vi "Tip tune ZaberAndSR865 Static.vi"(0 "Z axis":T3={"Serial port handle"="", "Axis"="", "Controller #"=0, "Min position"=0.0, "Max position"=0.0, "Min velocity"=0.0, "Max velocity"=0.0, "Firmware"="", "Device ID"=0, "Variable event"=refnum, "Variable ref"=refnum, "Resolution, usteps/step"=0, "Serial port semaphore"=refnum, "Joystick buttons"={"MinDir"=1, "MaxDir"=2, "MedSpeed"=5, "HighSpeed"=6}} {"Joystick buttons"."HighSpeed" min=1 max=25 step=1; "Joystick buttons"."MedSpeed" min=1 max=25 step=1; "Joystick buttons"."MaxDir" min=1 max=25 step=1; "Joystick buttons"."MinDir" min=1 max=25 step=1}, 1 "SR865":T1, 5 "error in":errorcluster) -> (19 "error out":errorcluster)   [LabVIEW 2018]
uses:
  Zaber library/Zaber.ctl
  GenericDataEvent/GenericEvent.ctl
  Zaber library/ZaberVariables.ctl
  SR865/SR865.ctl
  SR865/OutSineReference.ctl
  SR865/OutSineSource.ctl
  SR865/DataChannel.ctl
  <vilib>/Analysis/6fits.llb/Curve Fitting Criteria.ctl
  <vilib>/Analysis/NI_AAL_SigProc.lvlib
  <vilib>/Analysis/NI_AALBase.lvlib
  <vilib>/Analysis/NI_AALPro.lvlib
panel:
  in  "BtnQuit":bool
  in  "btnReadSignal":bool
  out "Signal":dbl=100000.0 caption="Signal, mV"
  in  "BtnZ-":bool
  in  "BtnZ+":bool
  in  "ZStep":dbl=0.005 caption="Z step, mm" min=0.0 max=25.0 step=0.01 format="%#.4f"
  in  "btnStartPosScanning":bool caption="stop"
  in  "btnCalculateSlope":bool
  in  "btnCalculateSurfaceLevel":bool
  in  "btnCalculateAirLevel":bool
  out "FrequencyStepRb":dbl=100000.0 caption="Frequency"
  out "PhaseRb":dbl=100000.0 caption="Frequency"
  out "AmplitudeRb":dbl=100000.0 caption="Frequency"
  out "DCOffsetRb":dbl=100000.0 caption="DC offset, V"
  out "SlopeError":dbl=8.6 caption="Slope error, V/mm" min=0.0 max=25.0 step=0.01 format="%#.4f"
  out "SurfaceError":dbl=8.6 caption="Surface error, V" min=0.0 max=25.0 step=0.01 format="%#.4f"
  out "AirError":dbl=8.6 caption="Air error, V" min=0.0 max=25.0 step=0.01 format="%#.4f"
  out "Slope":dbl=8.6 caption="Slope, mm/V" min=0.0 max=25.0 step=0.01 format="%#.4f"
  out "SurfaceLevel":dbl=8.6 caption="Surface level, V" min=0.0 max=25.0 step=0.01 format="%#.4f"
  out "AirLevel":dbl=8.6 caption="Air level, V" min=0.0 max=25.0 step=0.01 format="%#.4f"
  out "CurrentStep":i32=61 caption="Z steps"
  out "PltScanningPosition":cluster{dbl[], dbl[]}[](graph) caption="Position scanning"
  out "ZStep":dbl=0.0016666666666666607 caption="Z step, mm" min=0.0 max=25.0 format="%#.4f"
  in  "Frequency":dbl=97044.98 caption="Frequency, Hz" format="%.2p"
  in  "BtnSetZEndPosition":bool
  in  "BtnSetZStartPosition":bool
  in  "ZPoints":i32=61 caption="Z points"
  out "ZEndPosition":dbl=8.6 caption="Z end, mm" min=0.0 max=25.0 format="%#.4f"
  out "ZStartPosition":dbl=8.5 caption="Z start, mm" min=0.0 max=25.0 format="%#.4f"
  out "ZPositionRb":dbl=8.6 caption="Z position" min=0.0 max=25.0 step=0.01 format="%#.4f"
  in  "ZPosition":dbl=8.5 caption="Z position, mm" min=0.0 max=25.0 step=0.01 format="%#.4f"
  out "TblBestFrequencyies":string[][](table)=[["97044.98", "2.85"], ["82864.39", "1.68"], ["21141.21", "1.26"], ["93904.03", "0.82"], ["15778.11", "0.52"]] caption="Best frequencies, Hz"
  in  "TipPlace":u16(ring)=1 caption="Tip place" items=["Air", "Surface"]
  in  "SettingTime":u32=1000 caption="Setting time, ms"
  out "FrequencyRb":dbl=100000.0 caption="Frequency"
  out "CurrentPoint":i32=90
  out "PltScanningFrequence":cluster{dbl[], dbl[]}[](graph)=[{[10000.0, 11000.0, 12000.0, 13000.0, 14000.0, 15000.0, 16000.0, 17000.0, 18000.0, 19000.0, 20000.0, 21000.0, 22000.0, 23000.0, 24000.0, 25000.0, 26000.0, 27000.0, 28000.0, 29000.0, 30000.0, 31000.0, 32000.0, 33000.0, 34000.0, 35000.0, 36000.0, 37000.0, 38000.0, 39000.0, 40000.0, 41000.0, 42000.0, 43000.0, 44000.0, 45000.0, 46000.0, 47000.0, 48000.0, 49000.0, 50000.0, 51000.0, 52000.0, 53000.0, 54000.0, 55000.0, 56000.0, 57000.0, 58000.0, 59000.0, 60000.0, 61000.0, 62000.0, 63000.0, 64000.0, 65000.0, 66000.0, 67000.0, 68000.0, 69000.0, 70000.0, 71000.0, 72000.0, 73000.0, 74000.0, 75000.0, 76000.0, 77000.0, 78000.0, 79000.0, 80000.0, 81000.0, 82000.0, 83000.0, 84000.0, 85000.0, 86000.0, 87000.0, 88000.0, 89000.0, 90000.0, 91000.0, 92000.0, 93000.0, 94000.0, 95000.0, 96000.0, 97000.0, 98000.0, 99000.0, 100000.0], [3.5655190000512516, 3.4374305005139005, 3.4273711461139715, 3.4850248112142093, 3.5761130550998383, 3.556590231281875, 3.5082421792498932, 3.012145327734691, 3.60479334690102, 3.6237170567298436, 3.5213679819034964, 4.863866373270507, 4.004233765623082, 3.958662171251218, 3.638372868429504, 3.6863311988676024, 3.6407628928169347, 3.597268956374069, 3.472475578654757, 3.4138362740831423, 4.023460288827825, 3.8711427099095466, 3.8072787456116726, 3.773067870768127, 3.802872335674139, 3.843425482975206, 3.8131604010931146, 3.710485915669144, 3.68892415072003, 3.7175819077370553, 3.6497045488279003, 3.698426272759254, 3.738228894609222, 3.7572105957332433, 3.841541162636644, 3.552982648310411, 3.6359506328697484, 3.7367182179969376, 3.817937233155462, 3.940743403433729, 4.337961900873752, 3.232249392203631, 3.031809835447508, 3.1009883283630275, 3.1785447948663723, 2.9738534939166783, 3.794967857187948, 3.786370846678634, 3.691365712894553, 3.655859990170908, 3.6562916119155986, 3.5957679438322634, 3.593065477052433, 3.5925726553448727, 3.5922634338806207, 3.590250273321926, 3.597758557035468, 3.5946888897478324, 3.606027010467748, 3.573291409437125, 3.5650938203985896, 3.532467740941366, 3.385655269781037, 3.651862657728945, 3.6418741576807374, 3.5802843235408948, 3.611222575631784, 3.5164236610651676, 4.632535226763082, 3.2424697969441687, 3.272032610844888, 3.3549199729897623, 3.7972193768166784, 5.452081044437504, 2.748058067103696, 2.9130046647694234, 2.9576226283303546, 3.0336329490386387, 3.0499346821806705, 2.9810010016675736, 2.8330872460617447, 2.3801761264752517, 1.3887019949256822, 6.48560906859755, 5.721885978735551, 3.7523307011355125, 2.996072291328326, 5.390088024437564, 5.438011320322094, 4.595058047439225, 4.5440910275334865]}, {[10000.0, 11000.0, 12000.0, 13000.0, 14000.0, 15000.0, 16000.0, 17000.0, 18000.0, 19000.0, 20000.0, 21000.0, 22000.0, 23000.0, 24000.0, 25000.0, 26000.0, 27000.0, 28000.0, 29000.0, 30000.0, 31000.0, 32000.0, 33000.0, 34000.0, 35000.0, 36000.0, 37000.0, 38000.0, 39000.0, 40000.0, 41000.0, 42000.0, 43000.0, 44000.0, 45000.0, 46000.0, 47000.0, 48000.0, 49000.0, 50000.0, 51000.0, 52000.0, 53000.0, 54000.0, 55000.0, 56000.0, 57000.0, 58000.0, 59000.0, 60000.0, 61000.0, 62000.0, 63000.0, 64000.0, 65000.0, 66000.0, 67000.0, 68000.0, 69000.0, 70000.0, 71000.0, 72000.0, 73000.0, 74000.0, 75000.0, 76000.0, 77000.0, 78000.0, 79000.0, 80000.0, 81000.0, 82000.0, 83000.0, 84000.0, 85000.0, 86000.0, 87000.0, 88000.0, 89000.0, 90000.0, 91000.0, 92000.0, 93000.0, 94000.0, 95000.0, 96000.0, 97000.0, 98000.0, 99000.0, 100000.0], [3.6968028657407785, 3.397109339181018, 3.567193952093816, 3.4622519508906793, 3.5945342790368535, 3.5386940424582525, 3.029648511216874, 3.7294031949868516, 3.854496267967221, 3.66608362794549, 3.6337442084525384, 3.622335223134029, 3.520269601833684, 3.625449985669437, 3.5996783070122036, 3.596367060420739, 3.6706800775467205, 3.6178547324397927, 3.494530145248237, 3.4783507835572123, 3.9798696462301795, 3.909521653058709, 3.84636309009401, 3.8283541416529783, 3.8855956102501024, 3.948232372330415, 3.8955390259265563, 3.7044271046719377, 3.6476140823855085, 3.685313344462496, 3.639751480735465, 3.690521795627914, 3.727960158953497, 3.75535848669949, 3.8145229094921054, 3.5935582988975963, 3.6440902453414807, 3.730672290482194, 3.7940627371494946, 3.884890197869988, 4.123519414820418, 5.233578709141258, 2.8898807738384256, 2.709737263826195, 3.650699858167375, 3.6058691787236263, 3.5725795559217843, 3.585563635600408, 3.5978873993164835, 3.6012115301523817, 3.545358407800998, 3.557833559064785, 3.5697611313701043, 3.5699866053317777, 3.5644109564113067, 3.568540350922504, 3.570524521787714, 3.5653418417511418, 3.5472878205078633, 3.566549737959607, 3.5284381997956884, 3.443283156254747, 3.726391503493266, 3.6588555739683373, 3.5487920538102036, 3.744426212291304, 3.774333747133092, 3.7278280955270975, 4.291694487008893, 3.381445353898666, 3.4274420088262834, 3.5326255726860984, 3.8970271568359123, 3.8148611207822927, 4.140697353288415, 3.4812175242568655, 3.7482206201906454, 2.959581027358073, 2.755453572987086, 2.842289778548217, 2.8230407994627473, 2.5397852639697267, 1.7720535165304037, 6.311279502338936, 4.911483553972613, 3.8801745664846505, 3.1735908186482717, 2.5479667164400683, 5.117117280660982, 5.956381695510879, 6.236143926446963]}, {[10000.0, 11000.0, 12000.0, 13000.0, 14000.0, 15000.0, 16000.0, 17000.0, 18000.0, 19000.0, 20000.0, 21000.0, 22000.0, 23000.0, 24000.0, 25000.0, 26000.0, 27000.0, 28000.0, 29000.0, 30000.0, 31000.0, 32000.0, 33000.0, 34000.0, 35000.0, 36000.0, 37000.0, 38000.0, 39000.0, 40000.0, 41000.0, 42000.0, 43000.0, 44000.0, 45000.0, 46000.0, 47000.0, 48000.0, 49000.0, 50000.0, 51000.0, 52000.0, 53000.0, 54000.0, 55000.0, 56000.0, 57000.0, 58000.0, 59000.0, 60000.0, 61000.0, 62000.0, 63000.0, 64000.0, 65000.0, 66000.0, 67000.0, 68000.0, 69000.0, 70000.0, 71000.0, 72000.0, 73000.0, 74000.0, 75000.0, 76000.0, 77000.0, 78000.0, 79000.0, 80000.0, 81000.0, 82000.0, 83000.0, 84000.0, 85000.0, 86000.0, 87000.0, 88000.0, 89000.0, 90000.0, 91000.0, 92000.0, 93000.0, 94000.0, 95000.0, 96000.0, 97000.0, 98000.0, 99000.0, 100000.0], [-0.131283865689527, 0.04032116133288266, -0.1398228059798443, 0.022772860323529986, -0.018421223937015174, 0.017896188823622428, 0.47859366803301917, -0.7172578672521608, -0.24970292106620118, -0.04236657121564624, -0.112376226549042, 1.2415311501364776, 0.4839641637893983, 0.3332121855817811, 0.03869456141730021, 0.08996413844686346, -0.029917184729785884, -0.02058577606572376, -0.02205456659347993, -0.06451450947407, 0.043590642597645335, -0.03837894314916257, -0.03908434448233722, -0.05528627088485116, -0.0827232745759634, -0.10480688935520899, -0.08237862483344172, 0.0060588109972061766, 0.04131006833452133, 0.03226856327455918, 0.009953068092435124, 0.007904477131339682, 0.01026873565572517, 0.0018521090337535462, 0.02701825314453865, -0.04057565058718504, -0.008139612471732338, 0.006045927514743532, 0.023874496005967583, 0.05585320556374107, 0.2144424860533345, -2.0013293169376274, 0.14192906160908247, 0.39125106453683234, -0.47215506330100254, -0.632015684806948, 0.2223883012661636, 0.2008072110782262, 0.09347831357806946, 0.05464846001852619, 0.1109332041146005, 0.037934384767478235, 0.02330434568232853, 0.022586050013094994, 0.027852477469314074, 0.021709922399422155, 0.02723403524775403, 0.029347047996690634, 0.05873918995988481, 0.006741671477517919, 0.03665562060290117, 0.08918458468661905, -0.3407362337122293, -0.006992916239392244, 0.09308210387053384, -0.16414188875040914, -0.16311117150130805, -0.2114044344619299, 0.3408407397541886, -0.13897555695449748, -0.15540939798139553, -0.17770559969633615, -0.09980778001923385, 1.6372199236552114, -1.392639286184719, -0.568212859487442, -0.7905979918602908, 0.07405192168056551, 0.2944811091935846, 0.13871122311935657, 0.010046446598997338, -0.15960913749447503, -0.3833515216047214, 0.1743295662586144, 0.8104024247629376, -0.12784386534913805, -0.17751852731994555, 2.842121307997496, 0.32089403966111174, -1.3613236480716537, -1.6920528989134764]}] caption="Frequence scanning"
  in  "btnStartFreqScanning":bool caption="stop"
  out "FrequencyPoints":i32=91 caption="Frequency points"
  in  "FrequencyStep":dbl=1000.0 caption="Frequency step, Hz"
  in  "EndFrequency":dbl=100000.0 caption="End frequency, Hz" format="%.2p"
  in  "Phase":dbl format="%.3f"
  in  "StartFrequency":dbl=10000.0 caption="Start frequency, Hz" format="%.2p"
  in  "Amplitude":dbl=0.5 caption="Amplitude p-p, V" min=0.0 max=10.0 format="%.3f"
  # "RS865 parameters"
  # "Z stage parameters"
  # "Scanning parameters"
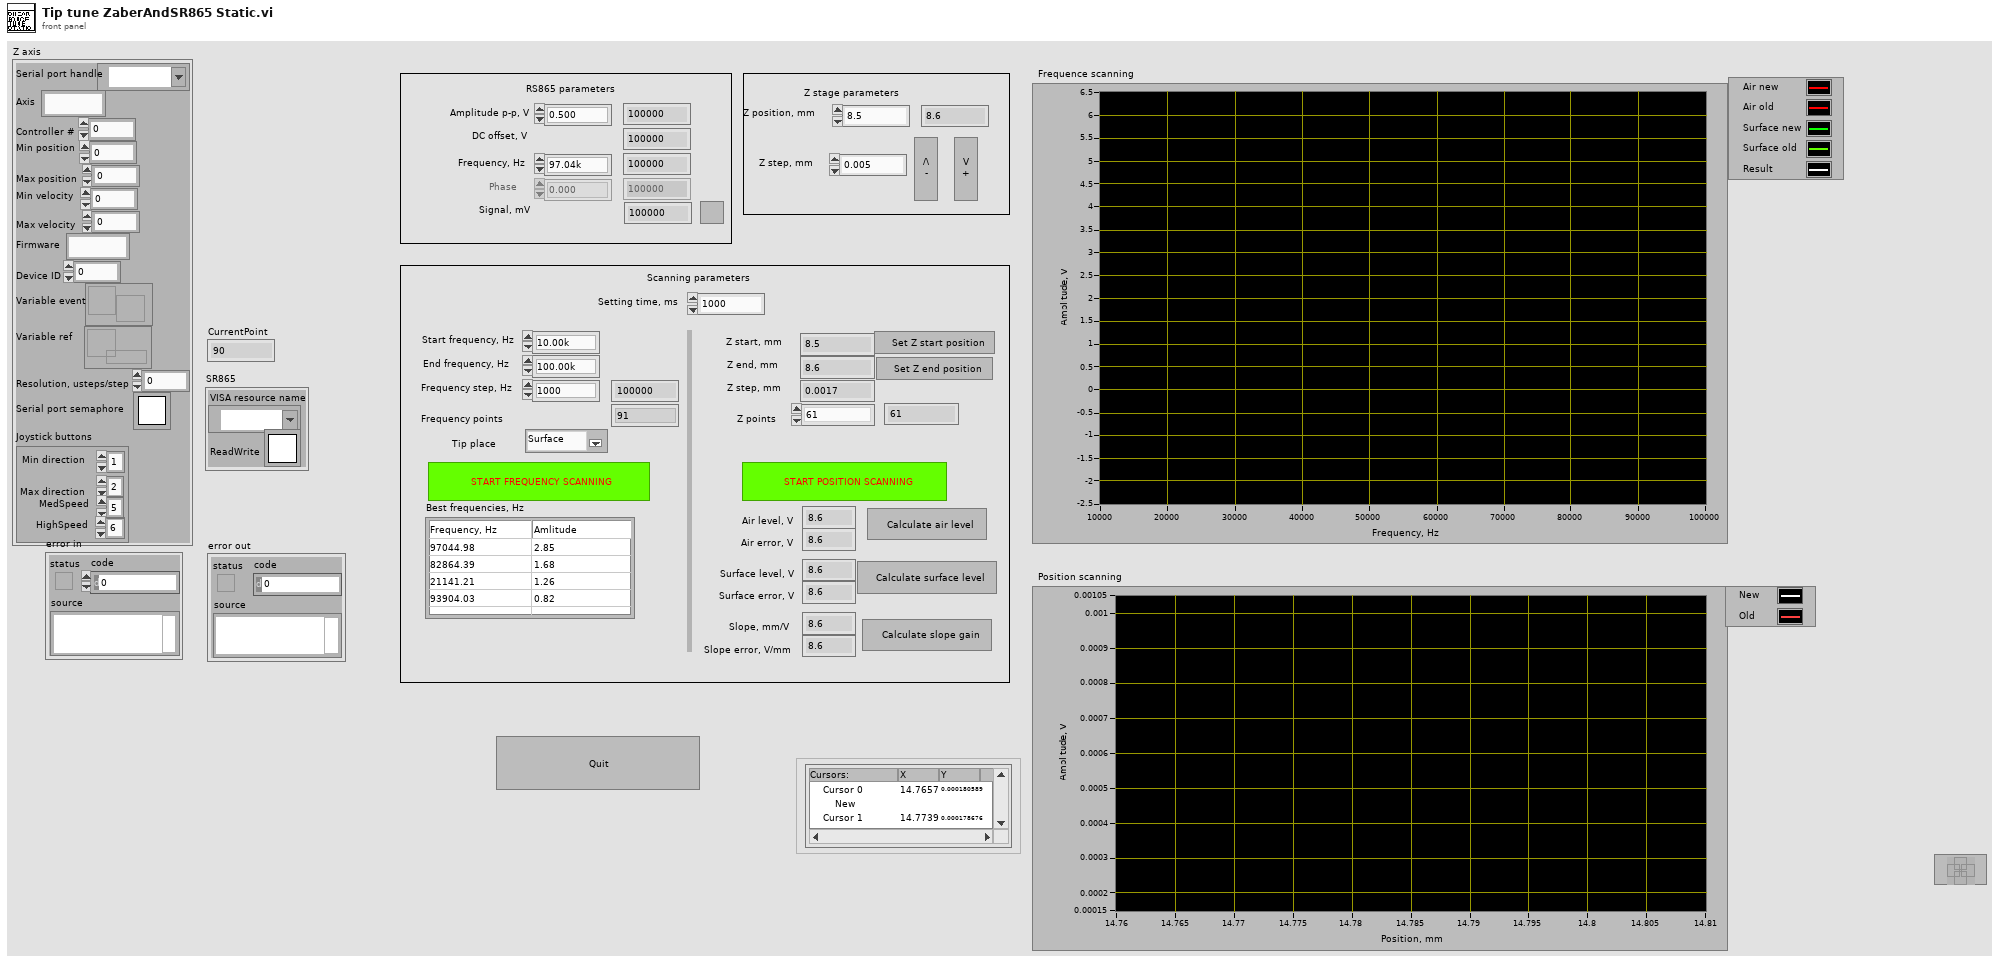
[diagram p1: front panel]
types:
  T1 = typedef "SR865.ctl" = cluster{"VISA resource name":refnum<visa-resource-name>, "ReadWrite":T2}
  T2 = typedef "Semaphore RefNum" = refnum<k1>
  T3 = typedef "Zaber.ctl" = cluster{"Serial port handle":refnum<visa-resource-name>, "Axis":string, "Controller #":u8, "Min position":dbl, "Max position":dbl, "Min velocity":dbl, "Max velocity":dbl, "Firmware":string, "Device ID":i32, "Variable event":T4, "Variable ref":refnum<data-value>, "Resolution, usteps/step":i32, "Serial port semaphore":T2, "Joystick buttons":cluster{"MinDir":i32, "MaxDir":i32, "MedSpeed":i32, "HighSpeed":i32}}
  T4 = typedef "GenericEvent.ctl" = refnum<user-event>
  T5 = typedef "DataChannel.ctl" = u16
  T6 = typedef "OutSineSource.ctl" = u16
  T7 = typedef "OutSineReference.ctl" = u16
  T8 = typedef "LVCursorListTypeDef.ctl" = cluster{"Name":string, "Color":u32, "Style":u8, "Point Style":u8, "Name Visible":bool, "Allow Drag":bool, "Cursor Mode":u32, "Plot":i32, "Index":i32, "Position":cluster{"X":dbl, "Y":dbl}, "X Scale":u32, "Y Scale":u32, "Watch Plots":i32[], "Watch All Plots":bool, "Plot Area":i32, "Label Offset":cluster{"X":dbl, "Y":dbl}}[]
  T9 = cluster{"Name":string, "Color":u32, "Style":u8, "Point Style":u8, "Name Visible":bool, "Allow Drag":bool, "Cursor Mode":u32, "Plot":i32, "Index":i32, "Position":cluster{"X":dbl, "Y":dbl}, "X Scale":u32, "Y Scale":u32, "Watch Plots":i32[], "Watch All Plots":bool, "Plot Area":i32, "Label Offset":cluster{"X":dbl, "Y":dbl}}
  T10 = typedef "NI_AALPro.lvlib/Curve Fitting Criteria.ctl" = u16
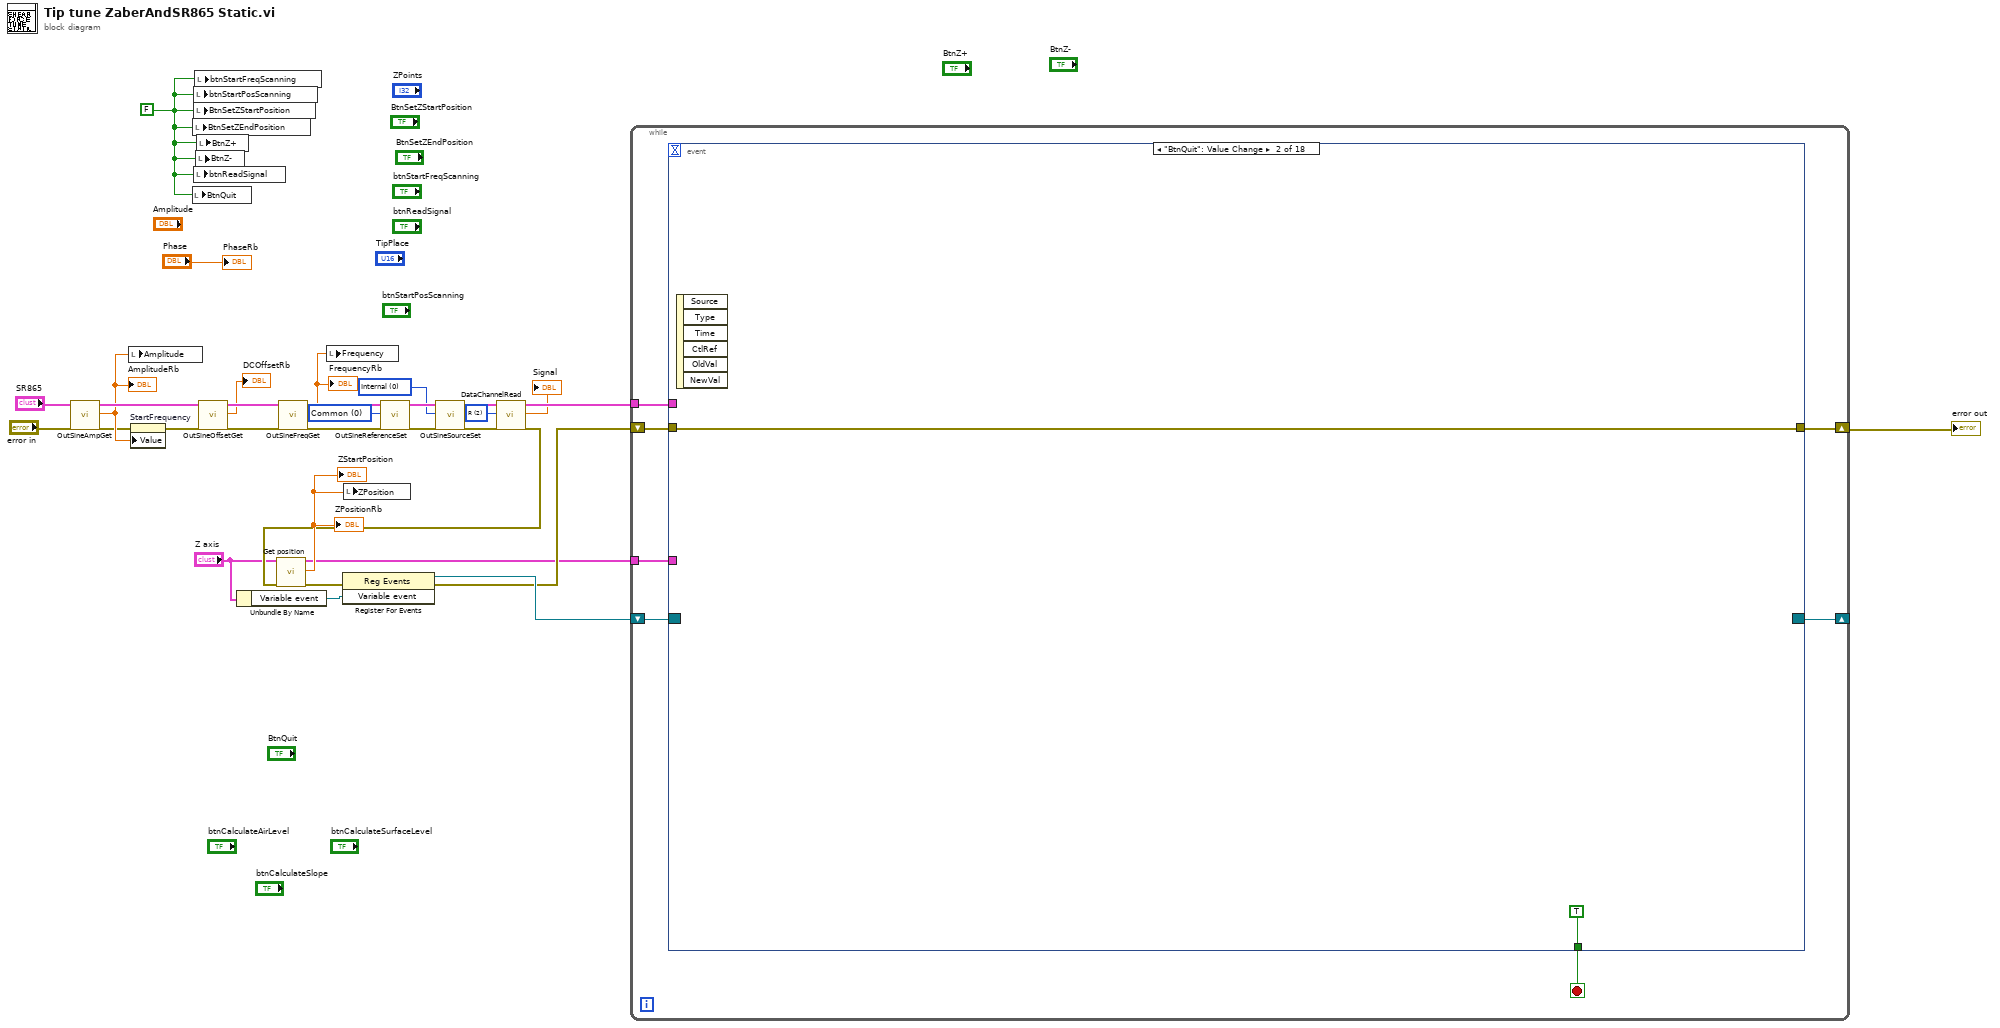
[diagram p0: block diagram]
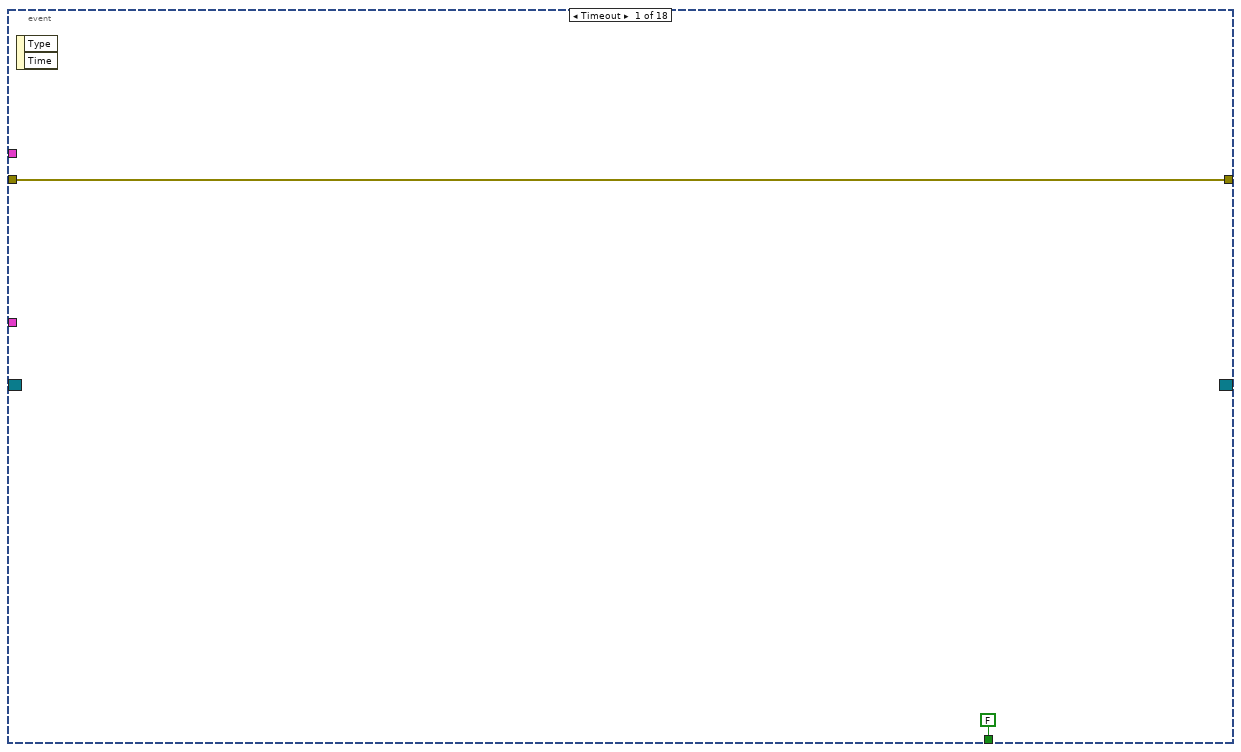
[diagram p2: hidden frame]
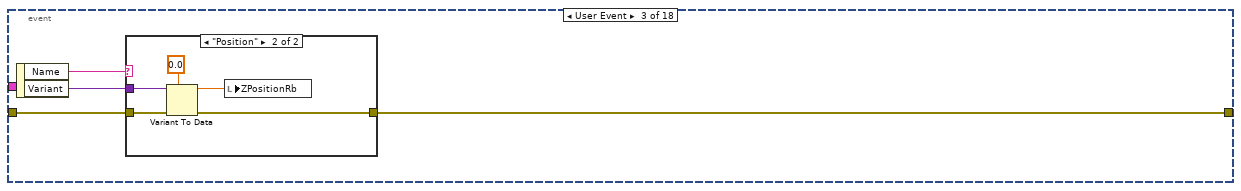
[diagram p3: hidden frame]
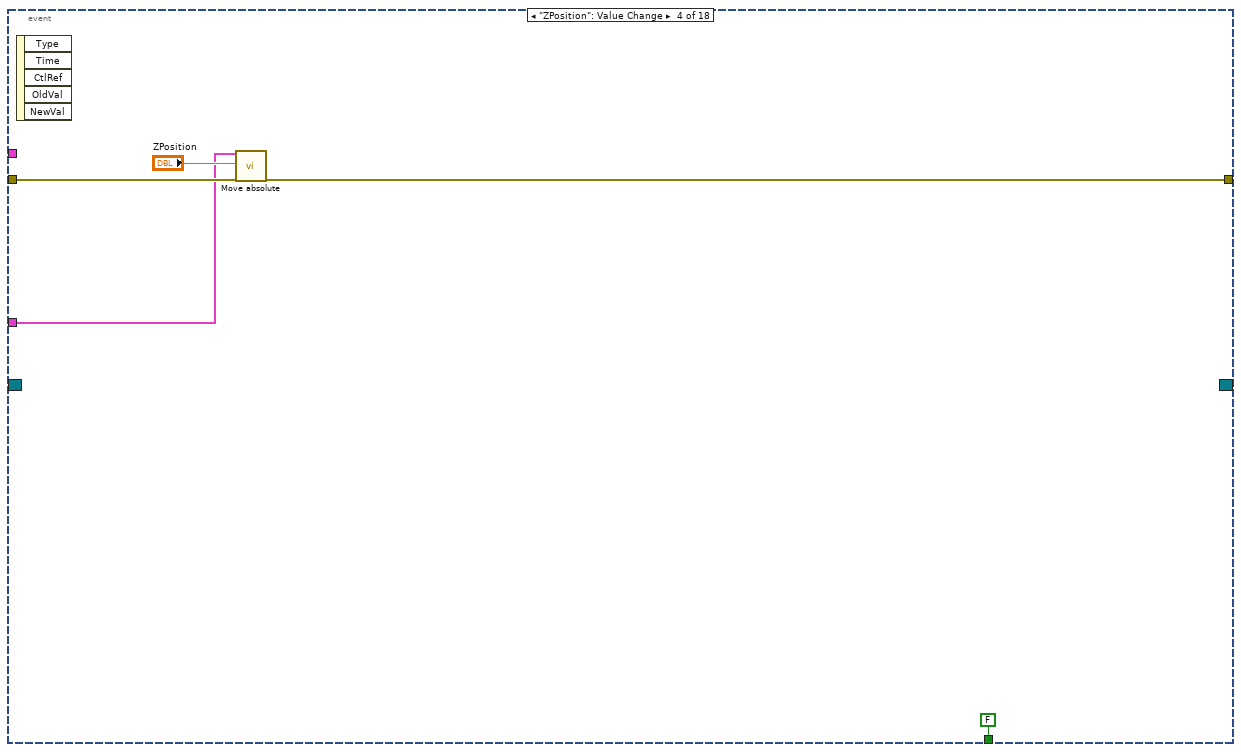
[diagram p5: hidden frame]
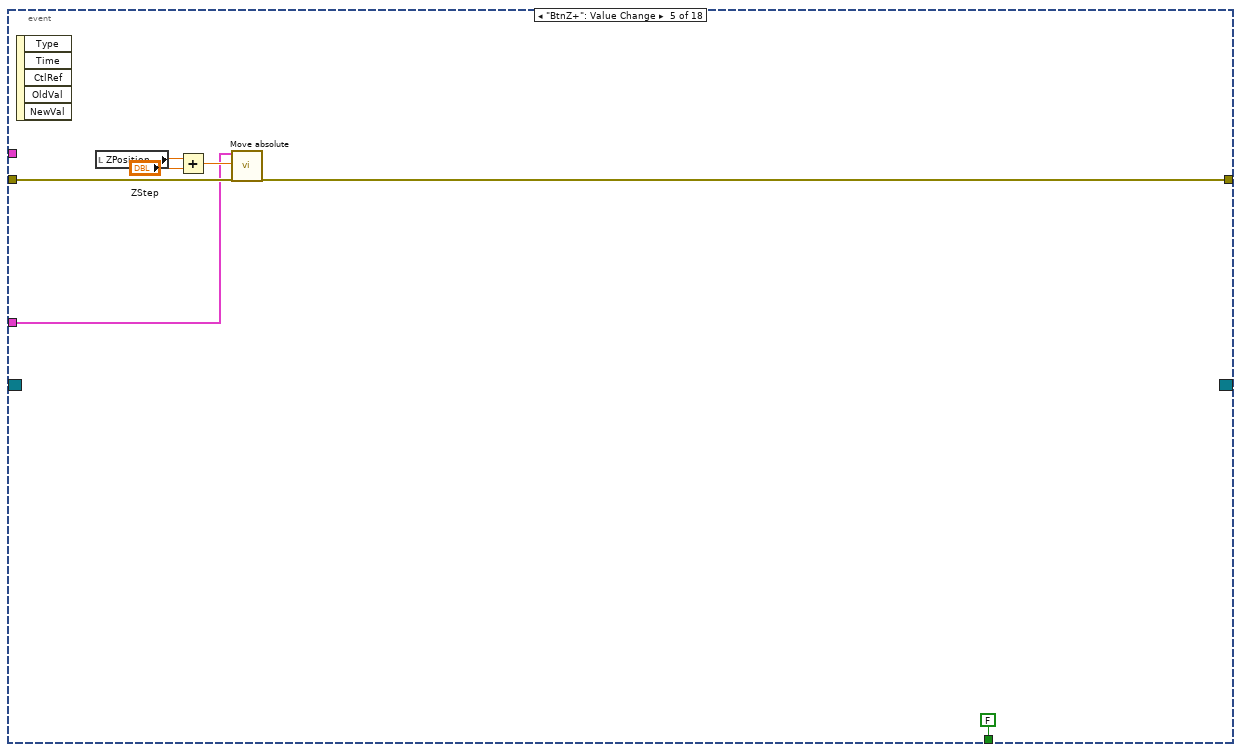
[diagram p6: hidden frame]
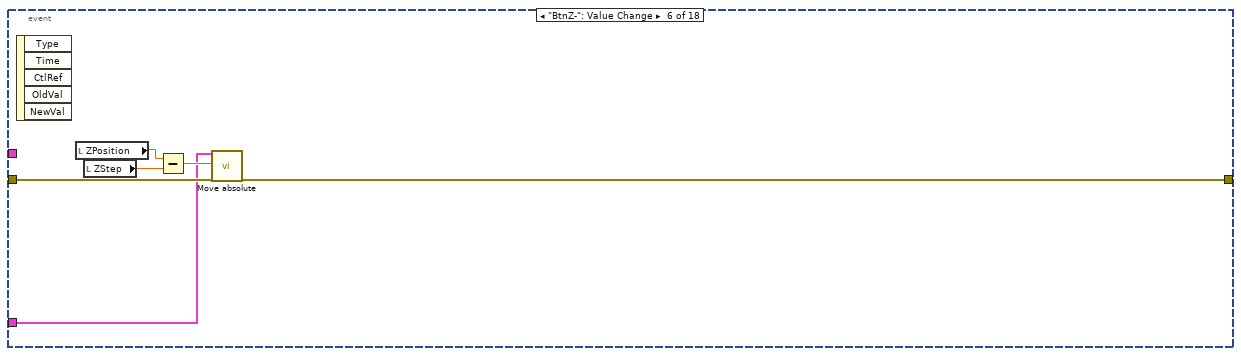
[diagram p7: hidden frame]
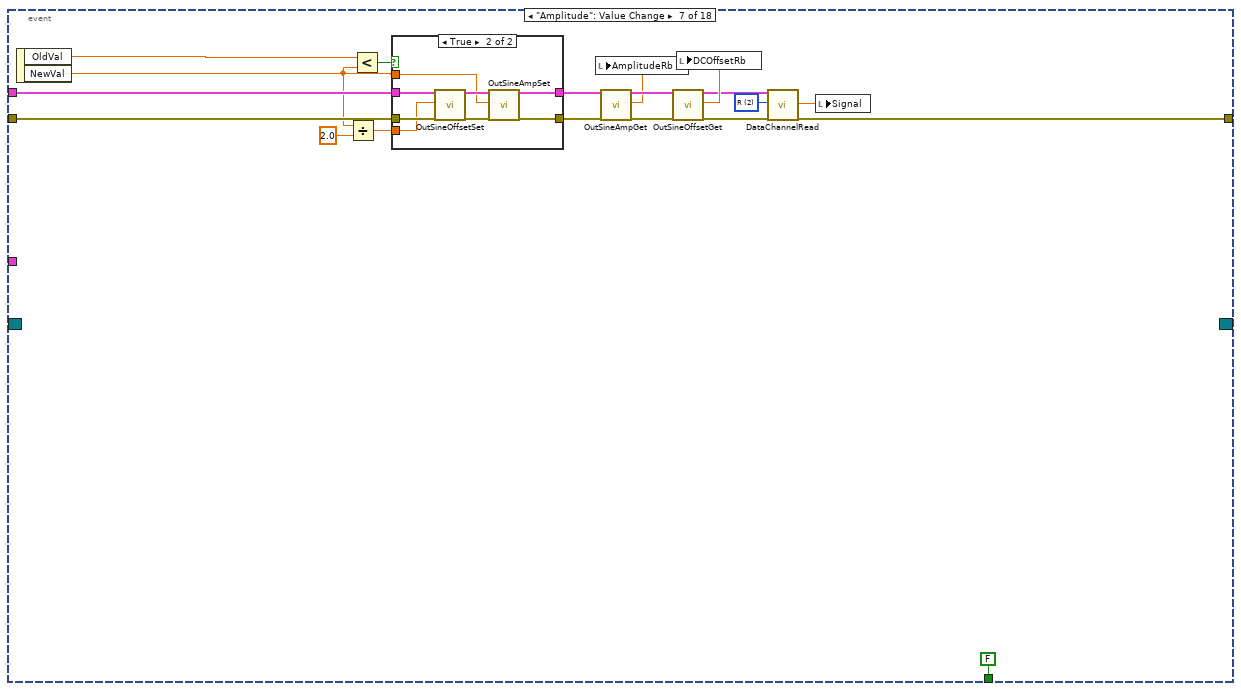
[diagram p8: hidden frame]
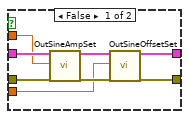
[diagram p9: hidden frame]
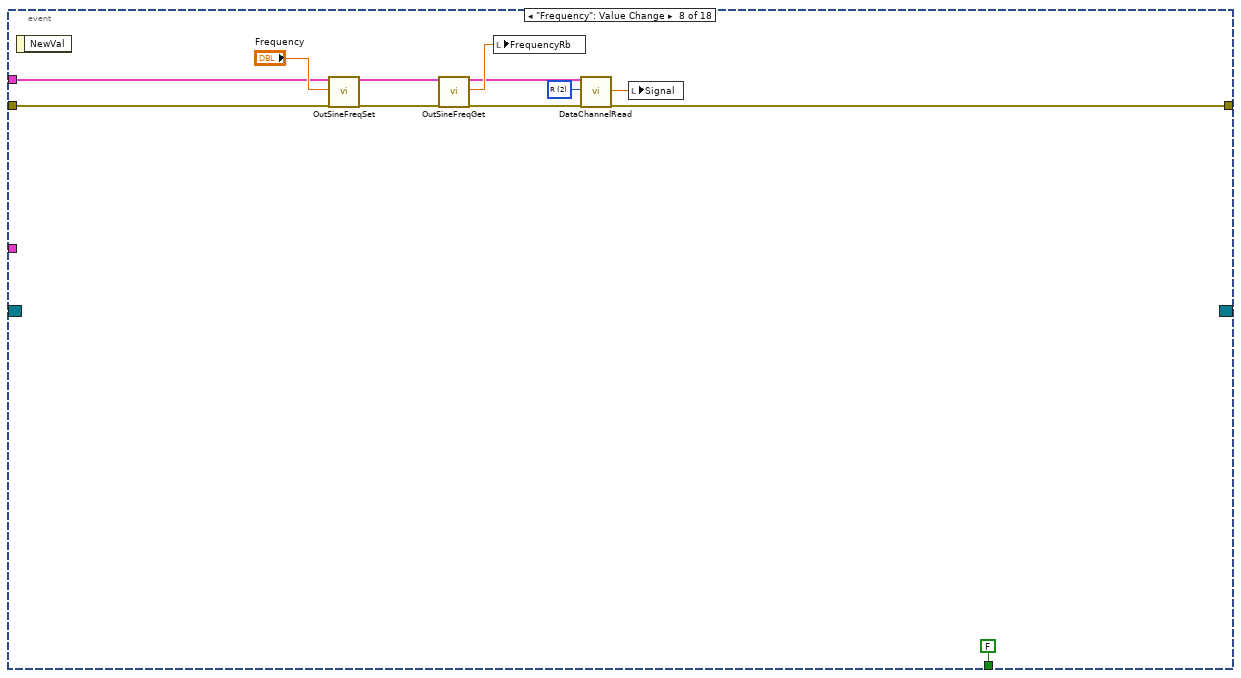
[diagram p10: hidden frame]
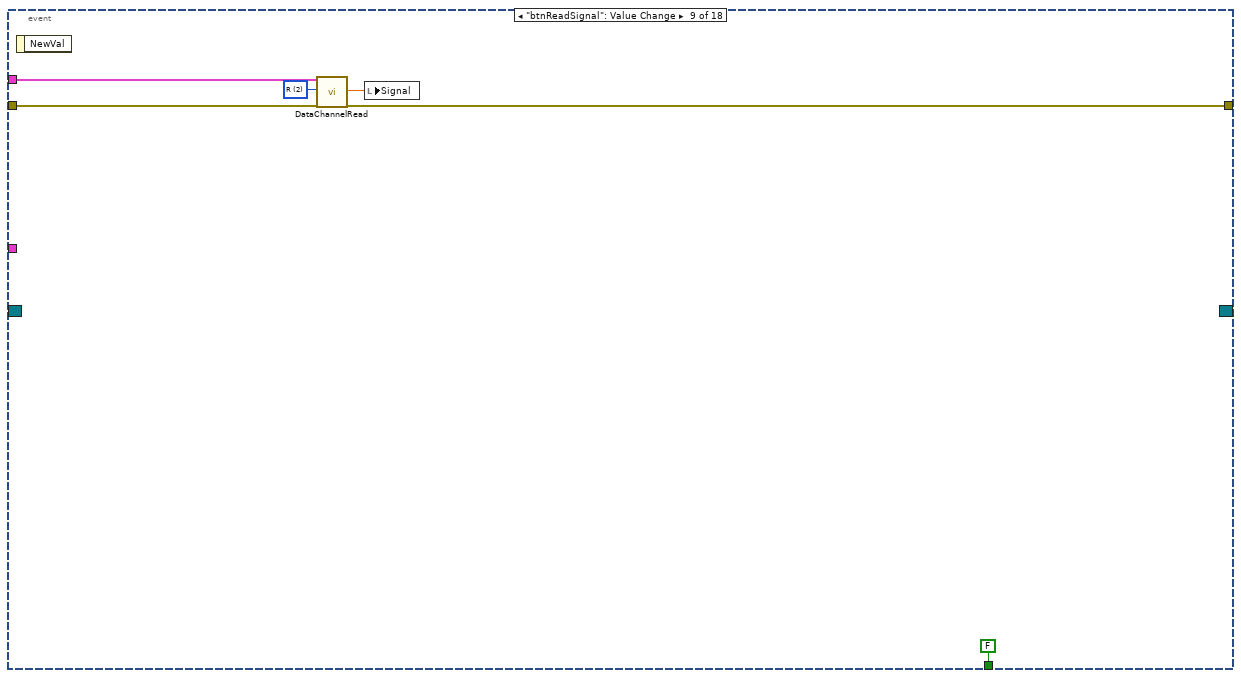
[diagram p11: hidden frame]
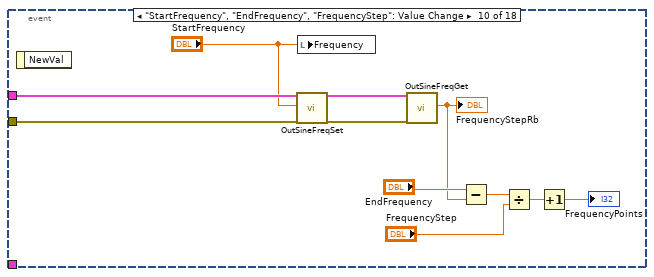
[diagram p12: hidden frame]
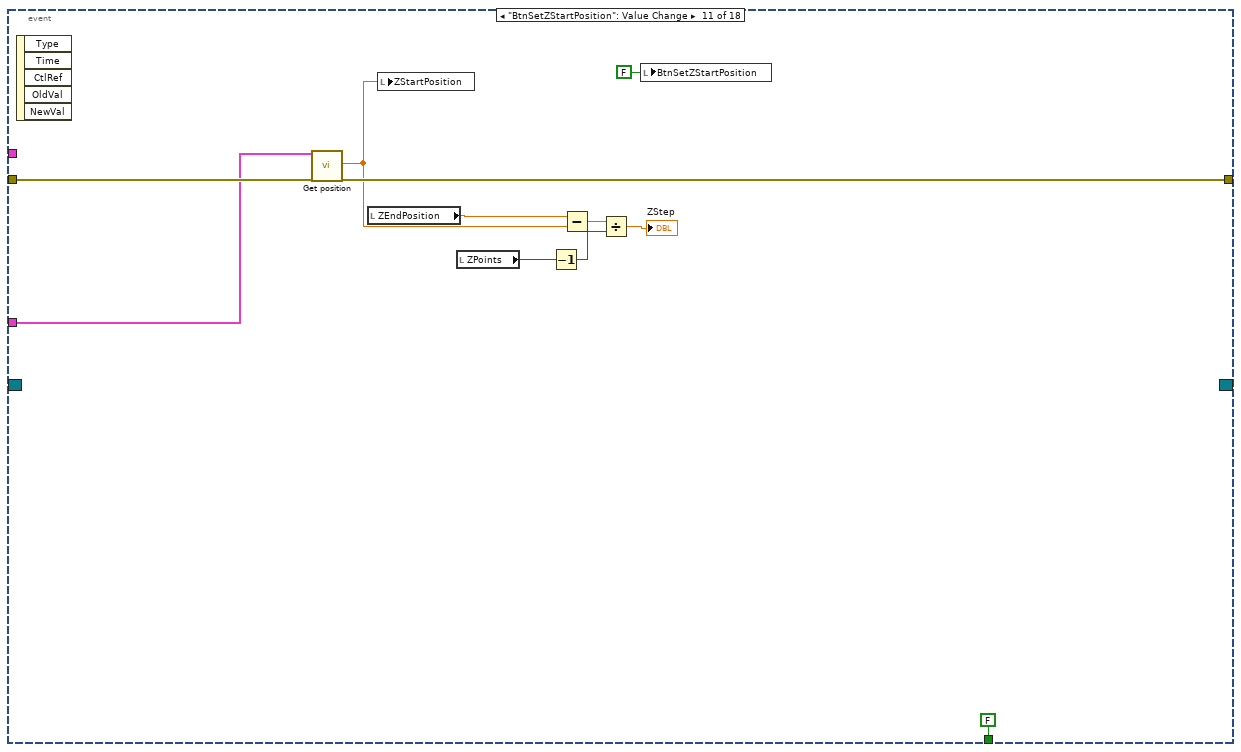
[diagram p13: hidden frame]
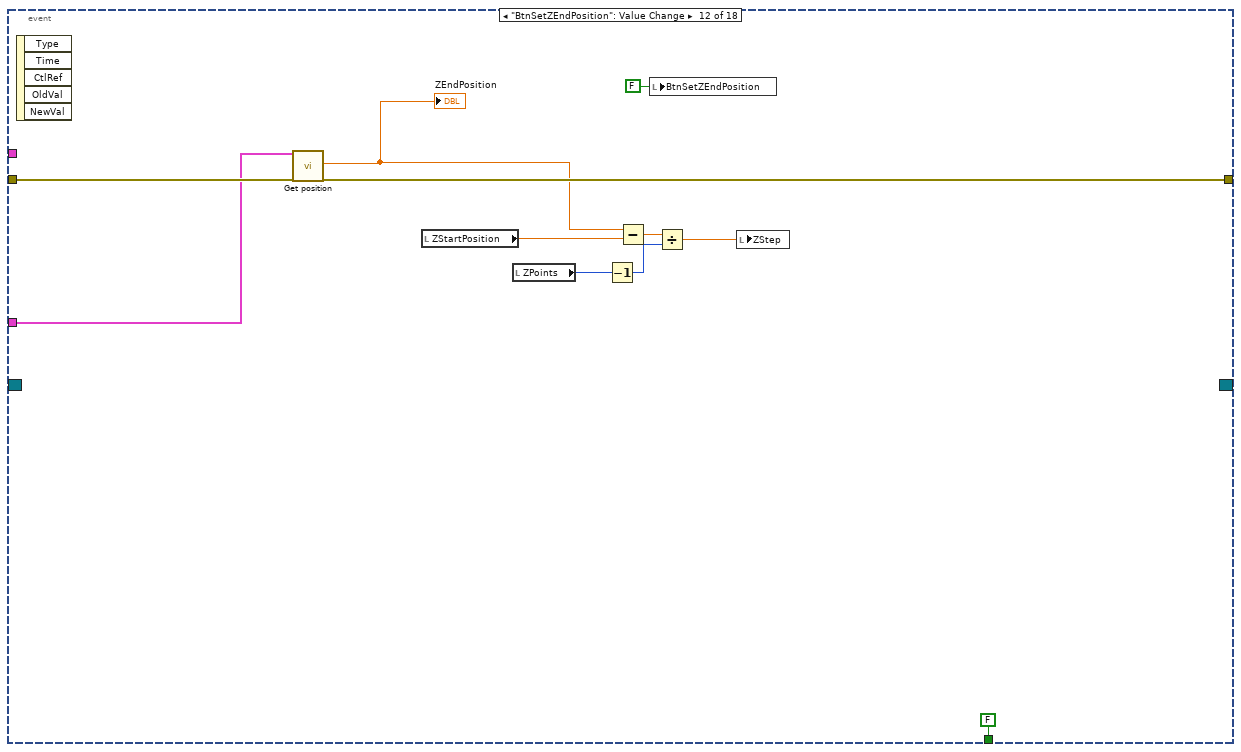
[diagram p14: hidden frame]
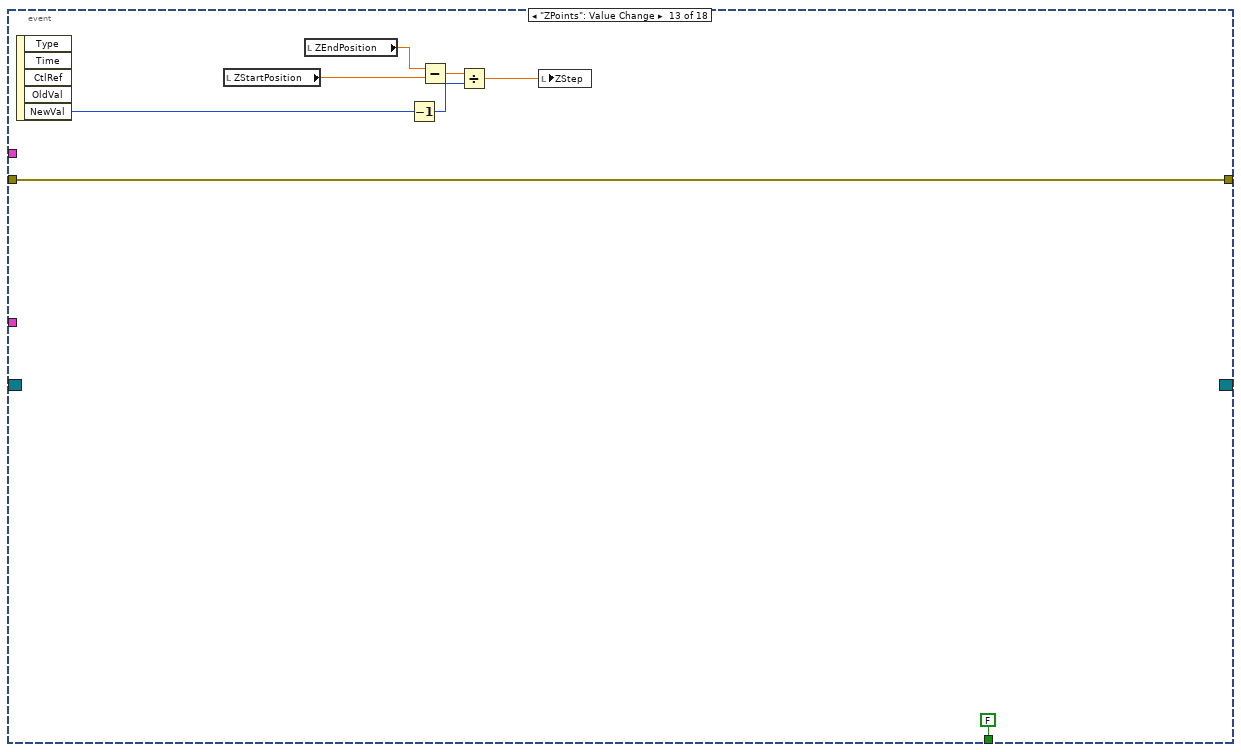
[diagram p15: hidden frame]
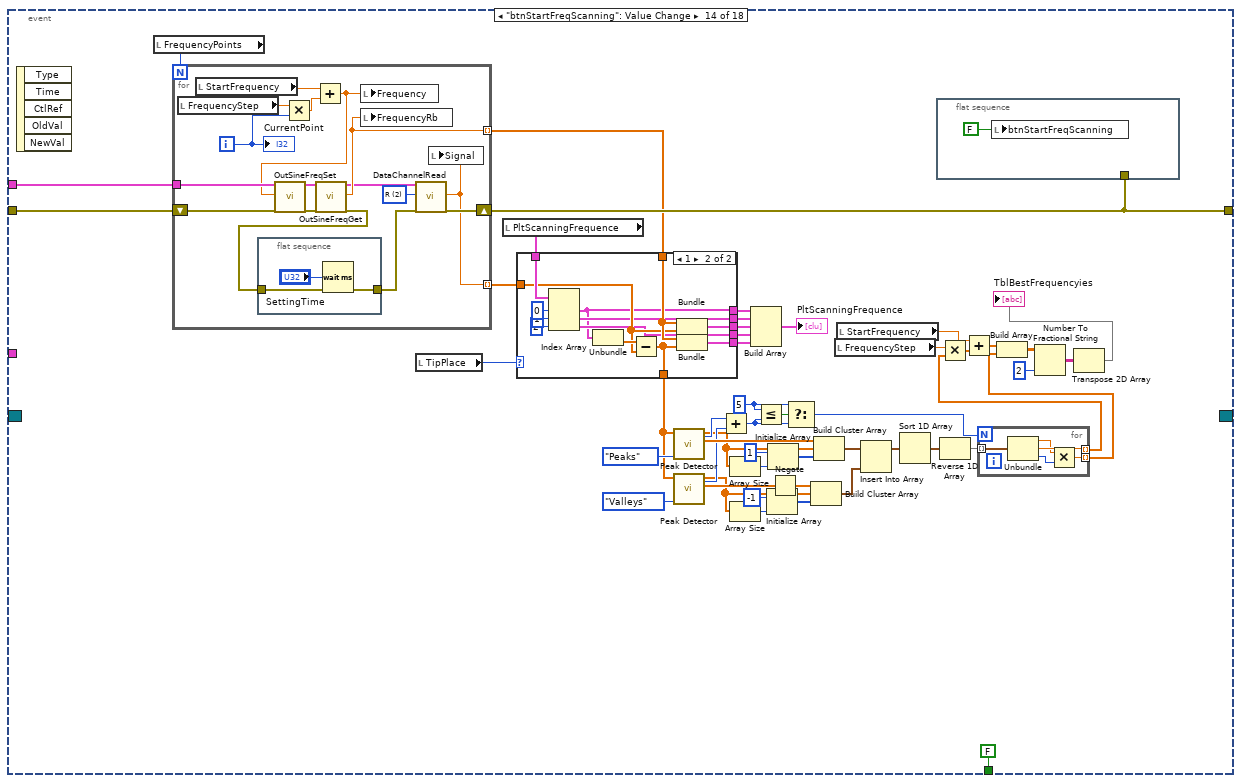
[diagram p16: hidden frame]
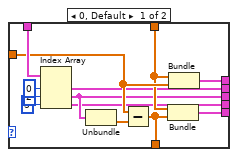
[diagram p17: hidden frame]
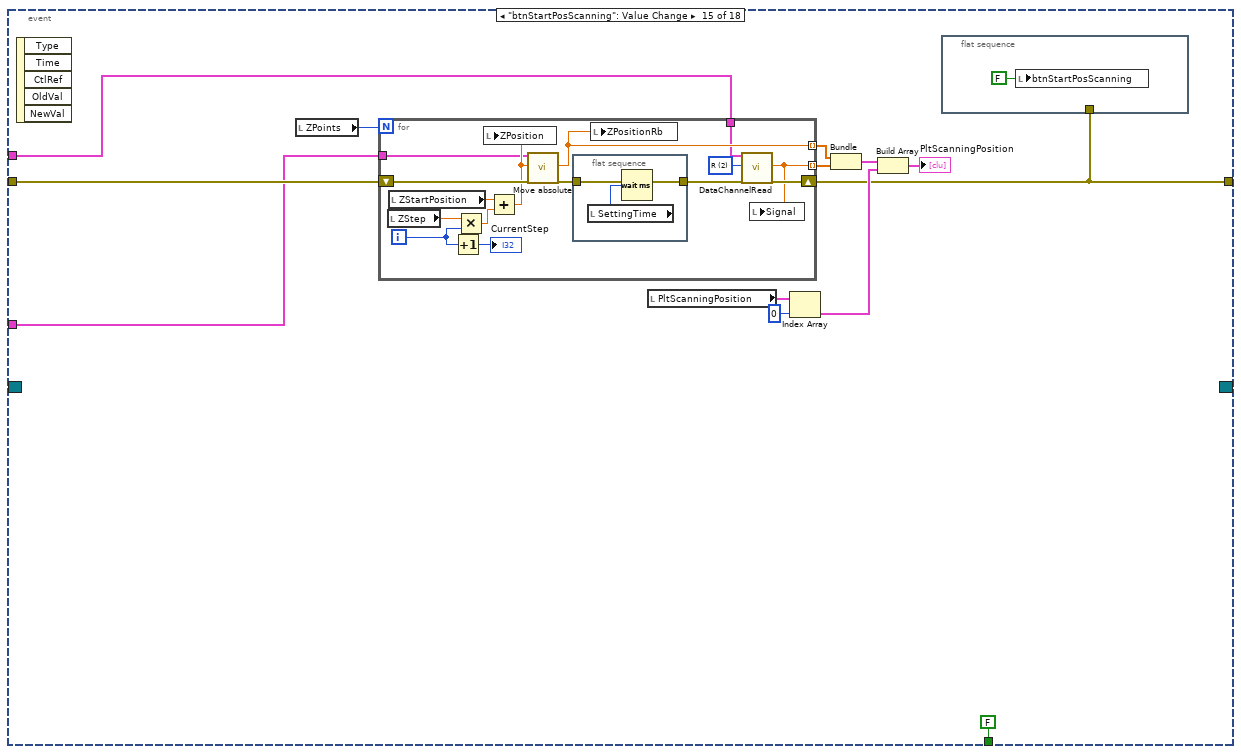
[diagram p18: hidden frame]
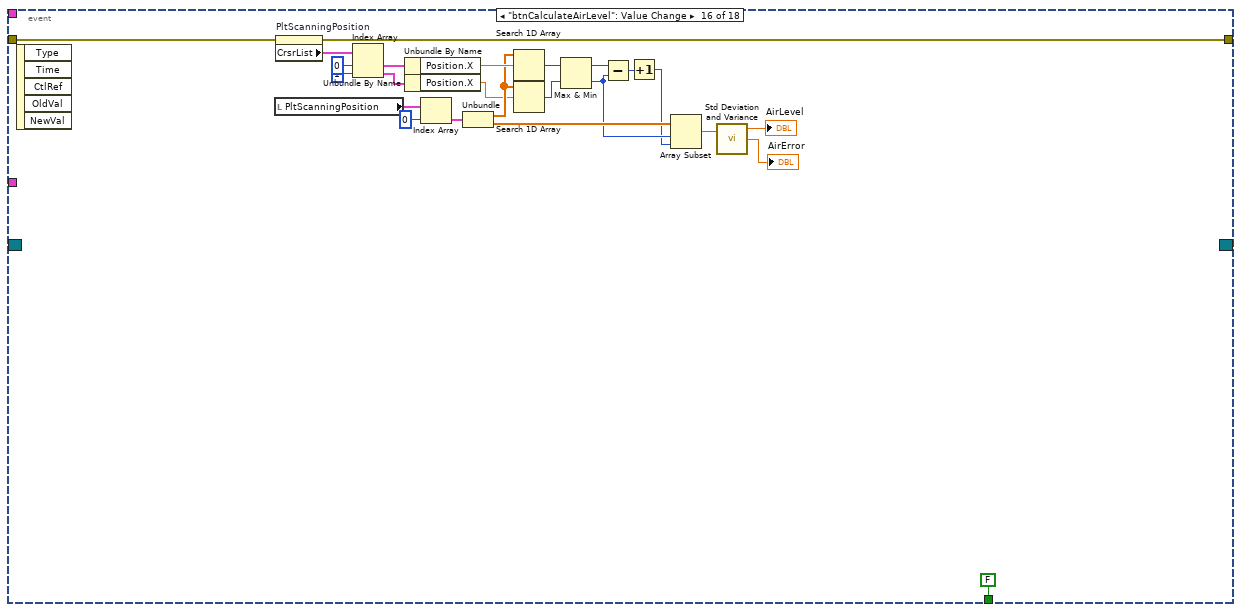
[diagram p19: hidden frame]
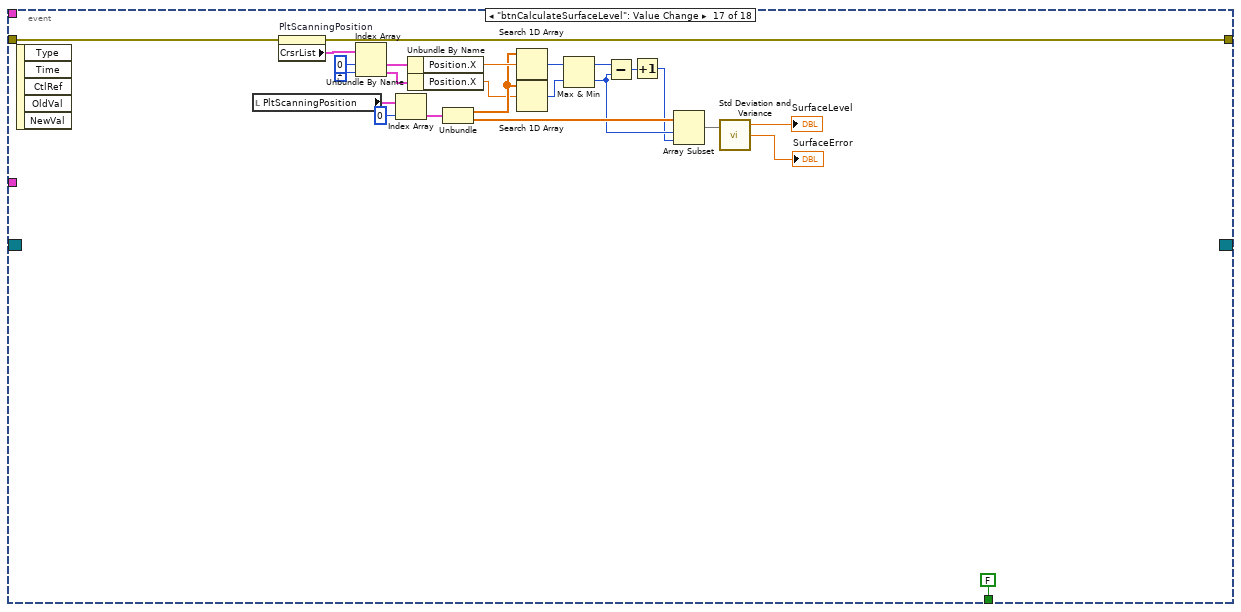
[diagram p20: hidden frame]
diagram:
  w12 = T5 2 items=["X", "Y", "R", "Theta", "IN1", "IN2", "IN3", "IN4", "OUT1", "OUT2", "XNoise", "YNoise", "Phase", "SineOut", "DCLevel", "IntRefFreq", "ExtRefFreq"] ("DataChannel")
  w20 = T6 0 items=["Internal", "External", "Dual", "Chop"] ("OutSineSource")
  w23 = T7 0 items=["Common", "Difference"] ("OutSineRef")
  w1 = FALSE ("btnStartStop")
  n1 = call "OutSineAmpGet.vi"("SR865 in"="SR865", "error in"="error in") -> ("SR865 out"=w30:T1, "Amplitude"=w17:dbl, "error out"=w16:errorcluster)  [unwired: 15 in]
  "AmplitudeRb" <- w17
  n2 = local write "Amplitude"(w17) -> ()
  n3 = property on="StartFrequency" class="DigNum (strict)"(error in=w16, "Value"=w17) -> (error out=w15:errorcluster)  [unwired: 1 in, 1 out]
  n4 = local write "BtnQuit"(w1) -> ()
  n5 = local write "BtnSetZEndPosition"(w1) -> ()
  n6 = local write "btnStartPosScanning"(w1) -> ()
  n7 = local write "BtnSetZStartPosition"(w1) -> ()
  n8 = local write "btnReadSignal"(w1) -> ()
  n9 = local write "btnStartFreqScanning"(w1) -> ()
  n10 = local write "BtnZ-"(w1) -> ()
  n11 = local write "BtnZ+"(w1) -> ()
  n12 = call "OutSineOffsetGet.vi"("SR865 in"=w30, "error in"=w15) -> ("SR865 out"=w29:T1, "Offset"=→"DCOffsetRb":dbl, "error out"=w28:errorcluster)  [unwired: 15 in]
  n13 = Unbundle By Name("Z axis") -> ("Variable event"=w2:T4)
  n14 = call "OutSineFreqGet.vi"("SR865 in"=w29, "error in"=w28) -> ("SR865 out"=w24:T1, "Frequency"=w13:dbl, "error out"=w25:errorcluster)  [unwired: 15 in]
  "FrequencyRb" <- w13
  n15 = local write "Frequency"(w13) -> ()
  n16 = call "OutSineReferenceSet.vi"("SR865 in"=w24, "OutSineRef"=w23, "error in"=w25) -> ("SR865 out"=w21:T1, "error out"=w22:errorcluster)  [unwired: 15 in]
  n17 = call "OutSineSourceSet.vi"("SR865 in"=w21, "OutSineSource"=w20, "error in"=w22) -> ("SR865 out"=w10:T1, "error out"=w11:errorcluster)  [unwired: 15 in]
  n18 = call "DataChannelRead.vi"("SR865 in"=w10, "DataChannel"=w12, "error in"=w11) -> ("SR865 out"=w9:T1, "Signal"=→"Signal":dbl, "error out"=w6:errorcluster)  [unwired: 14 in]
  n19 = call "Get position.vi"("Zaber"="Z axis", "error in"=w6) -> ("Zaber out"=w4:T3, "PositionRb"=w14:dbl, "error out"=w5:errorcluster)  [unwired: 13 in, 2 out]
  "ZPositionRb" <- w14
  "ZStartPosition" <- w14
  n20 = register-events(error in=w5, w2) -> (reference out=w32:refnum<event-registration>, error out=w18:errorcluster)  [unwired: 1 in]
  n21 = local write "ZPosition"(w14) -> ()
  n22 = while {
    tunnel: w9 -> [w39]
    tunnel: w4 -> [w36]
    shift-right: [w37] -> w7
    shift-left: w18 -> [w38]
    shift-right: [w33] -> _
    shift-left: w32 -> [w35]
    stop <- w34 stop-if-true
    n23 = event shown="[1] \"BtnQuit\": Value Change" {
      selector: w35 -> [_ _ _ _ _ _ _ _ _ _ _ _ _ _ _ _ _ _]
      dyn-events: [_ _ _ _ _ _ _ _ _ _ _ _ _ _ _ _ _ _] -> w33
      timeout: _ -> [_ _ _ _ _ _ _ _ _ _ _ _ _ _ _ _ _ _]
      tunnel: w39 -> [_ _ _ _ _ _ w88 w117 w122 w133 _ _ _ w215 w269 _ _ _]
      tunnel: w38 -> [w41 w42 w47 w57 w65 w69 w89 w116 w123 w132 w140 w151 w158 w214 w270 w302 w326 w350]
      tunnel: [w41 w42 w46 w56 w61 w68 w73 w108 w120 _ w139 w150 w158 w212 w266 w301 w325 w349] -> w37
      tunnel: w36 -> [_ _ _ w54 w59 w66 _ _ _ _ w136 w147 _ _ w268 _ _ _]
      tunnel: [FALSE TRUE _ FALSE FALSE _ FALSE FALSE FALSE _ FALSE FALSE FALSE FALSE FALSE FALSE FALSE FALSE] -> w34
      event Timeout {
        n24 = event-data() -> ()  [unwired: 1 in, 2 out]
      }
      event "BtnQuit": Value Change {
        n25 = event-data() -> ()  [unwired: 1 in, 6 out]
      }
      event User Event {
        n26 = event-data() -> ("Name"=w44:string, "Variant"=w45:variant)  [unwired: 1 in]
        n27 = case shown="\"Position\"" w44 {
          tunnel: w47 -> [w48 w51]
          tunnel: [w48 w50] -> w46
          tunnel: w45 -> [_ w49]
          frame Default {
          }
          frame "Position" {
            n28 = Variant To Data(error in=w51, type=0.0, Variant=w49) -> (data=w52:dbl, error out=w50:errorcluster)
            n29 = local write "ZPositionRb"(w52) -> ()
          }
        }
      }
      event "ZPosition": Value Change {
        n30 = event-data() -> ()  [unwired: 1 in, 5 out]
        n31 = call "Move absolute.vi"("Zaber"=w54, "Position, mm"="ZPosition", "error in"=w57) -> ("error out"=w56:errorcluster)  [unwired: 13 in, 3 out]
      }
      event "BtnZ+": Value Change {
        n32 = event-data() -> ()  [unwired: 1 in, 5 out]
        n33 = local read "ZPosition"() -> (w64:dbl)
        n34 = Add(x=w64, y="ZStep") -> (x+y=w62:dbl)
        n35 = call "Move absolute.vi"("Zaber"=w59, "Position, mm"=w62, "error in"=w65) -> ("error out"=w61:errorcluster)  [unwired: 13 in, 3 out]
      }
      event "BtnZ-": Value Change {
        n36 = event-data() -> ()  [unwired: 1 in, 5 out]
        n37 = local read "ZPosition"() -> (w71:dbl)
        n38 = local read "ZStep"() -> (w67:dbl)
        n39 = Subtract(x=w71, y=w67) -> (x-y=w70:dbl)
        n40 = call "Move absolute.vi"("Zaber"=w66, "Position, mm"=w70, "error in"=w69) -> ("error out"=w68:errorcluster)  [unwired: 13 in, 3 out]
      }
      event "Amplitude": Value Change {
        w76 = T5 2 items=["X", "Y", "R", "Theta", "IN1", "IN2", "IN3", "IN4", "OUT1", "OUT2", "XNoise", "YNoise", "Phase", "SineOut", "DCLevel", "IntRefFreq", "ExtRefFreq"] ("DataChannel")
        n41 = event-data() -> ("OldVal"=w86:dbl, "NewVal"=w77:dbl)  [unwired: 1 in]
        n42 = Divide(x=w77, y=2.0) -> (x/y=w78:dbl)
        n43 = Less?(x=w86, y=w77) -> (x < y?=w87:bool)
        n44 = case shown="True" w87 {
          tunnel: w89 -> [w98 w106]
          tunnel: [w96 w104] -> w84
          tunnel: w88 -> [w95 w103]
          tunnel: [w93 w101] -> w82
          tunnel: w77 -> [w92 w100]
          tunnel: w78 -> [w91 w99]
          frame False {
            n45 = call "OutSineAmpSet.vi"("SR865 in"=w95, "Amplitude"=w92, "error in"=w98) -> ("SR865 out"=w94:T1, "error out"=w97:errorcluster)  [unwired: 15 in]
            n46 = call "OutSineOffsetSet.vi"("SR865 in"=w94, "Amplitude"=w91, "error in"=w97) -> ("SR865 out"=w93:T1, "error out"=w96:errorcluster)  [unwired: 15 in]
          }
          frame True {
            n47 = call "OutSineOffsetSet.vi"("SR865 in"=w103, "Amplitude"=w99, "error in"=w106) -> ("SR865 out"=w102:T1, "error out"=w105:errorcluster)  [unwired: 15 in]
            n48 = call "OutSineAmpSet.vi"("SR865 in"=w102, "Amplitude"=w100, "error in"=w105) -> ("SR865 out"=w101:T1, "error out"=w104:errorcluster)  [unwired: 15 in]
          }
        }
        n49 = call "OutSineAmpGet.vi"("SR865 in"=w82, "error in"=w84) -> ("SR865 out"=w83:T1, "Amplitude"=w80:dbl, "error out"=w85:errorcluster)  [unwired: 15 in]
        n50 = local write "AmplitudeRb"(w80) -> ()
        n51 = call "OutSineOffsetGet.vi"("SR865 in"=w83, "error in"=w85) -> ("SR865 out"=w72:T1, "Offset"=w81:dbl, "error out"=w74:errorcluster)  [unwired: 15 in]
        n52 = local write "DCOffsetRb"(w81) -> ()
        n53 = call "DataChannelRead.vi"("SR865 in"=w72, "DataChannel"=w76, "error in"=w74) -> ("Signal"=w75:dbl, "error out"=w73:errorcluster)  [unwired: 14 in, 1 out]
        n54 = local write "Signal"(w75) -> ()
      }
      event "Frequency": Value Change {
        w111 = T5 2 items=["X", "Y", "R", "Theta", "IN1", "IN2", "IN3", "IN4", "OUT1", "OUT2", "XNoise", "YNoise", "Phase", "SineOut", "DCLevel", "IntRefFreq", "ExtRefFreq"] ("DataChannel")
        n55 = event-data() -> ()  [unwired: 1 in, 1 out]
        n56 = call "OutSineFreqSet.vi"("SR865 in"=w117, "Frequency"="Frequency", "error in"=w116) -> ("SR865 out"=w114:T1, "error out"=w115:errorcluster)  [unwired: 15 in]
        n57 = call "OutSineFreqGet.vi"("SR865 in"=w114, "error in"=w115) -> ("SR865 out"=w107:T1, "Frequency"=w113:dbl, "error out"=w109:errorcluster)  [unwired: 15 in]
        n58 = local write "FrequencyRb"(w113) -> ()
        n59 = call "DataChannelRead.vi"("SR865 in"=w107, "DataChannel"=w111, "error in"=w109) -> ("Signal"=w110:dbl, "error out"=w108:errorcluster)  [unwired: 14 in, 1 out]
        n60 = local write "Signal"(w110) -> ()
      }
      event "btnReadSignal": Value Change {
        w124 = T5 2 items=["X", "Y", "R", "Theta", "IN1", "IN2", "IN3", "IN4", "OUT1", "OUT2", "XNoise", "YNoise", "Phase", "SineOut", "DCLevel", "IntRefFreq", "ExtRefFreq"] ("DataChannel")
        n61 = event-data() -> ()  [unwired: 1 in, 1 out]
        n62 = call "DataChannelRead.vi"("SR865 in"=w122, "DataChannel"=w124, "error in"=w123) -> ("Signal"=w121:dbl, "error out"=w120:errorcluster)  [unwired: 14 in, 1 out]
        n63 = local write "Signal"(w121) -> ()
      }
      event "StartFrequency", "EndFrequency", "FrequencyStep": Value Change {
        n64 = event-data() -> ()  [unwired: 1 in, 1 out]
        n65 = call "OutSineFreqSet.vi"("SR865 in"=w133, "Frequency"="StartFrequency", "error in"=w132) -> ("SR865 out"=w134:T1, "error out"=w135:errorcluster)  [unwired: 15 in]
        n66 = local write "Frequency"("StartFrequency") -> ()
        n67 = call "OutSineFreqGet.vi"("SR865 in"=w134, "error in"=w135) -> ("Frequency"=w125:dbl)  [unwired: 15 in, 2 out]
        "FrequencyStepRb" <- w125
        n68 = Subtract(x="EndFrequency", y=w125) -> (x-y=w130:dbl)
        n69 = Divide(x=w130, y="FrequencyStep") -> (x/y=w128:dbl)
        n70 = Increment(x=w128) -> (x+1=→"FrequencyPoints":dbl)
      }
      event "BtnSetZStartPosition": Value Change {
        n71 = event-data() -> ()  [unwired: 1 in, 5 out]
        n72 = call "Get position.vi"("Zaber"=w136, "error in"=w140) -> ("PositionRb"=w137:dbl, "error out"=w139:errorcluster)  [unwired: 13 in, 3 out]
        n73 = local read "ZEndPosition"() -> (w142:dbl)
        n74 = local write "ZStartPosition"(w137) -> ()
        n75 = local read "ZPoints"() -> (w144:i32)
        n76 = Decrement(x=w144) -> (x-1=w143:i32)
        n77 = Subtract(x=w142, y=w137) -> (x-y=w145:dbl)
        n78 = Divide(x=w145, y=w143) -> (x/y=→"ZStep":dbl)
        n79 = local write "BtnSetZStartPosition"(FALSE ("BtnSetZStartPosition")) -> ()
      }
      event "BtnSetZEndPosition": Value Change {
        n80 = event-data() -> ()  [unwired: 1 in, 5 out]
        n81 = call "Get position.vi"("Zaber"=w147, "error in"=w151) -> ("PositionRb"=w149:dbl, "error out"=w150:errorcluster)  [unwired: 13 in, 3 out]
        "ZEndPosition" <- w149
        n82 = local read "ZStartPosition"() -> (w153:dbl)
        n83 = local read "ZPoints"() -> (w155:i32)
        n84 = Decrement(x=w155) -> (x-1=w154:i32)
        n85 = Subtract(x=w149, y=w153) -> (x-y=w156:dbl)
        n86 = local write "BtnSetZEndPosition"(FALSE ("BtnSetZEndPosition")) -> ()
        n87 = Divide(x=w156, y=w154) -> (x/y=w152:dbl)
        n88 = local write "ZStep"(w152) -> ()
      }
      event "ZPoints": Value Change {
        n89 = event-data() -> ("NewVal"=w160:i32)  [unwired: 1 in, 4 out]
        n90 = local read "ZStartPosition"() -> (w163:dbl)
        n91 = local read "ZEndPosition"() -> (w161:dbl)
        n92 = Decrement(x=w160) -> (x-1=w164:i32)
        n93 = Subtract(x=w161, y=w163) -> (x-y=w165:dbl)
        n94 = Divide(x=w165, y=w164) -> (x/y=w162:dbl)
        n95 = local write "ZStep"(w162) -> ()
      }
      event "btnStartFreqScanning": Value Change {
        w206 = 5
        n96 = event-data() -> ()  [unwired: 1 in, 5 out]
        n97 = local read "FrequencyPoints"() -> (w211:i32)
        n98 = for {
          N: w211 -> [_]
          tunnel: w215 -> [w254]
          tunnel: [w252] -> w175 mode=indexing
          tunnel: [w247] -> w210 mode=indexing
          shift-right: [w251] -> w212
          shift-left: w214 -> [w256]
          i -> [w261]
          w248 = T5 2 items=["X", "Y", "R", "Theta", "IN1", "IN2", "IN3", "IN4", "OUT1", "OUT2", "XNoise", "YNoise", "Phase", "SineOut", "DCLevel", "IntRefFreq", "ExtRefFreq"] ("DataChannel")
          n99 = local read "FrequencyStep"() -> (w262:dbl)
          n100 = local read "StartFrequency"() -> (w259:dbl)
          n101 = flat-sequence {
            tunnel: w255 -> [w263]
            tunnel: [w263] -> w249
            frame #0 {
              n102 = Wait (ms)(milliseconds to wait="SettingTime") -> ()  [unwired: 1 out]
            }
          }
          n103 = Multiply(x=w262, y=w261) -> (x*y=w260:dbl)
          n104 = Add(x=w259, y=w260) -> (x+y=w253:dbl)
          n105 = call "OutSineFreqSet.vi"("SR865 in"=w254, "Frequency"=w253, "error in"=w256) -> ("SR865 out"=w257:T1, "error out"=w258:errorcluster)  [unwired: 15 in]
          n106 = call "OutSineFreqGet.vi"("SR865 in"=w257, "error in"=w258) -> ("SR865 out"=w250:T1, "Frequency"=w252:dbl, "error out"=w255:errorcluster)  [unwired: 15 in]
          n107 = local write "Frequency"(w253) -> ()
          n108 = local write "FrequencyRb"(w252) -> ()
          n109 = call "DataChannelRead.vi"("SR865 in"=w250, "DataChannel"=w248, "error in"=w249) -> ("Signal"=w247:dbl, "error out"=w251:errorcluster)  [unwired: 14 in, 1 out]
          n110 = local write "Signal"(w247) -> ()
          "CurrentPoint" <- w261
        }
        n111 = local read "TipPlace"() -> (w167:u16)
        n112 = local read "PltScanningFrequence"() -> (w209:cluster{dbl[], dbl[]}[])
        n113 = case shown="1" w167 {
          tunnel: w210 -> [w230 w240]
          tunnel: w209 -> [w232 w245]
          tunnel: w175 -> [w228 w243]
          tunnel: [w227 w242] -> w174
          tunnel: [w225 w235] -> w173
          tunnel: [w224 w237] -> w172
          tunnel: [w223 w239] -> w171
          tunnel: [w222 w236] -> w170
          tunnel: [w221 w234] -> w169
          frame 0, Default {
            n114 = Index Array(array=w232, index #1=0 ("index"), index #2=2 ("index"), index #3=3 ("index")) -> (element #1=w224:cluster{dbl[], dbl[]}, element #2=w223:cluster{dbl[], dbl[]}, element #3=w222:cluster{dbl[], dbl[]})
            n115 = Unbundle(w223) -> (w229:dbl[])  [unwired: 1 out]
            n116 = Subtract(x=w230, y=w229) -> (x-y=w227:dbl[])
            n117 = Bundle(w228, w227) -> (w221:cluster{dbl[], dbl[]})  [unwired: 1 in]
            n118 = Bundle(w228, w230) -> (w225:cluster{dbl[], dbl[]})  [unwired: 1 in]
          }
          frame 1 {
            n119 = Index Array(array=w245, index #1=0 ("index"), index #2=1 ("index"), index #3=2 ("index")) -> (element #1=w235:cluster{dbl[], dbl[]}, element #2=w237:cluster{dbl[], dbl[]}, element #3=w236:cluster{dbl[], dbl[]})
            n120 = Unbundle(w235) -> (w241:dbl[])  [unwired: 1 out]
            n121 = Subtract(x=w241, y=w240) -> (x-y=w242:dbl[])
            n122 = Bundle(w243, w240) -> (w239:cluster{dbl[], dbl[]})  [unwired: 1 in]
            n123 = Bundle(w243, w242) -> (w234:cluster{dbl[], dbl[]})  [unwired: 1 in]
          }
        }
        n124 = call <vilib>:"Peak Detector.vi"("peaks/valleys"=enum32{"Peaks", "Valleys"}."Peaks", "X"=w174) -> ("Amplitudes"=w198:dbl[], "Locations"=w187:dbl[], "# found"=w190:i32)  [unwired: 5 in, 2 out]
        n125 = call <vilib>:"Peak Detector.vi"("peaks/valleys"=enum32{"Peaks", "Valleys"}."Valleys", "X"=w174) -> ("Amplitudes"=w183:dbl[], "Locations"=w181:dbl[], "# found"=w191:i32)  [unwired: 5 in, 2 out]
        n126 = Add(x=w190, y=w191) -> (x+y=w189:i32)
        n127 = Array Size(array=w187) -> (size(s)=w186:i32)
        n128 = Array Size(array=w181) -> (size(s)=w184:i32)
        n129 = Build Array(w173, w172, w171, w170, w169) -> (→"PltScanningFrequence":cluster{dbl[], dbl[]}[])
        n130 = Less Or Equal?(x=w206, y=w189) -> (x <= y?=w207:bool)
        n131 = Initialize Array(-1, w184) -> (w179:i32[])
        n132 = Initialize Array(1, w186) -> (w180:i32[])
        n133 = Negate(x=w183) -> (-x=w182:dbl[])
        n134 = Select(t=w206, s=w207, f=w189) -> (s? t:f=w197:i32)
        n135 = Build Cluster Array(w182, w181, w179) -> (w177:cluster{dbl, dbl, i32}[])
        n136 = Build Cluster Array(w198, w187, w180) -> (w178:cluster{dbl, dbl, i32}[])
        n137 = local read "FrequencyStep"() -> (w205:dbl)
        n138 = local read "StartFrequency"() -> (w203:dbl)
        n139 = Insert Into Array(array=w178, new element=w177) -> (w176:cluster{dbl, dbl, i32}[])  [unwired: 1 in]
        n140 = Sort 1D Array(array=w176) -> (sorted array=w193:cluster{dbl, dbl, i32}[])
        n141 = flat-sequence {
          tunnel: w212 -> [_]
          frame #0 {
            n142 = local write "btnStartFreqScanning"(FALSE ("btnStartStopScanningPosition")) -> ()
          }
        }
        n143 = Reverse 1D Array(array=w193) -> (reversed array=w194:cluster{dbl, dbl, i32}[])
        n144 = for {
          N: w197 -> [_]
          tunnel: w194 -> [w220] mode=indexing
          tunnel: [w218] -> w195 mode=indexing
          tunnel: [w216] -> w196 mode=indexing
          n145 = Unbundle(w220) -> (w217:dbl, w218:dbl, w219:i32)
          n146 = Multiply(x=w217, y=w219) -> (x*y=w216:dbl)
        }
        n147 = Multiply(x=w205, y=w195) -> (x*y=w204:dbl[])
        n148 = Add(x=w203, y=w204) -> (x+y=w202:dbl[])
        n149 = Build Array(w202, w196) -> (w201:dbl[][])
        n150 = Number To Fractional String(number=w201, precision (6)=i16 2) -> (F-format string=w199:string[][])  [unwired: 2 in]
        n151 = Transpose 2D Array(2D array=w199) -> (transposed array=→"TblBestFrequencyies":string[][])
      }
      event "btnStartPosScanning": Value Change {
        n152 = event-data() -> ()  [unwired: 1 in, 5 out]
        n153 = local read "ZPoints"() -> (w278:i32)
        n154 = for {
          N: w278 -> [_]
          tunnel: w268 -> [w280]
          shift-right: [w284] -> w266
          shift-left: w270 -> [w289]
          tunnel: [w287] -> w273 mode=indexing
          tunnel: [w281] -> w272 mode=indexing
          tunnel: w269 -> [w283]
          i -> [w290]
          w286 = T5 2 items=["X", "Y", "R", "Theta", "IN1", "IN2", "IN3", "IN4", "OUT1", "OUT2", "XNoise", "YNoise", "Phase", "SineOut", "DCLevel", "IntRefFreq", "ExtRefFreq"] ("DataChannel")
          n155 = local read "ZStep"() -> (w294:dbl)
          n156 = local read "ZStartPosition"() -> (w292:dbl)
          n157 = Increment(x=w290) -> (x+1=→"CurrentStep":i32)
          n158 = Multiply(x=w294, y=w290) -> (x*y=w293:dbl)
          n159 = Add(x=w292, y=w293) -> (x+y=w282:dbl)
          n160 = local write "ZPosition"(w282) -> ()
          n161 = call "Move absolute.vi"("Zaber"=w280, "Position, mm"=w282, "error in"=w289) -> ("Position, mm"=w287:dbl, "error out"=w288:errorcluster)  [unwired: 13 in, 2 out]
          n162 = flat-sequence {
            tunnel: [w296] -> w285
            tunnel: w288 -> [w296]
            frame #0 {
              n163 = local read "SettingTime"() -> (w295:u32)
              n164 = Wait (ms)(milliseconds to wait=w295) -> ()  [unwired: 1 out]
            }
          }
          n165 = local write "ZPositionRb"(w287) -> ()
          n166 = call "DataChannelRead.vi"("SR865 in"=w283, "DataChannel"=w286, "error in"=w285) -> ("Signal"=w281:dbl, "error out"=w284:errorcluster)  [unwired: 14 in, 1 out]
          n167 = local write "Signal"(w281) -> ()
        }
        n168 = local read "PltScanningPosition"() -> (w277:cluster{dbl[], dbl[]}[])
        n169 = Index Array(array=w277, index=0) -> (element=w276:cluster{dbl[], dbl[]})
        n170 = Bundle(w273, w272) -> (w271:cluster{dbl[], dbl[]})  [unwired: 1 in]
        n171 = Build Array(w271, w276) -> (→"PltScanningPosition":cluster{dbl[], dbl[]}[])
        n172 = flat-sequence {
          tunnel: w266 -> [_]
          frame #0 {
            n173 = local write "btnStartPosScanning"(FALSE ("btnStartPosScanning")) -> ()
          }
        }
      }
      event "btnCalculateAirLevel": Value Change {
        n174 = event-data() -> ()  [unwired: 1 in, 5 out]
        n175 = local read "PltScanningPosition"() -> (w300:cluster{dbl[], dbl[]}[])
        n176 = property on="PltScanningPosition" class="XYGraph (strict)"(error in=w302) -> (error out=w301:errorcluster, "CrsrList"=w320:T8)  [unwired: 1 in, 1 out]
        n177 = Index Array(array=w320, index #1=0 ("index"), index #2=1 ("index")) -> (element #1=w317:T9, element #2=w316:T9)
        n178 = Unbundle By Name(w317) -> ("Position.X"=w315:dbl)
        n179 = Unbundle By Name(w316) -> ("Position.X"=w312:dbl)
        n180 = Index Array(array=w300, index=0) -> (element=w299:cluster{dbl[], dbl[]})
        n181 = Unbundle(w299) -> (w314:dbl[], w313:dbl[])
        n182 = Search 1D Array(1D array=w314, element=w315) -> (index of element=w311:i32)  [unwired: 1 in]
        n183 = Search 1D Array(1D array=w314, element=w312) -> (index of element=w310:i32)  [unwired: 1 in]
        n184 = Max & Min(x=w311, y=w310) -> (max(x,y)=w309:i32, min(x,y)=w308:i32)
        n185 = Subtract(x=w309, y=w308) -> (x-y=w307:i32)
        n186 = Increment(x=w307) -> (x+1=w306:i32)
        n187 = Array Subset(array=w313, index=w308, length=w306) -> (w305:dbl[])
        n188 = call <vilib>:"Std Deviation and Variance.vi"("X"=w305) -> ("mean"=→"AirLevel":dbl, "standard deviation"=→"AirError":dbl)  [unwired: 1 in, 1 out]
      }
      event "btnCalculateSurfaceLevel": Value Change {
        n189 = event-data() -> ()  [unwired: 1 in, 5 out]
        n190 = local read "PltScanningPosition"() -> (w324:cluster{dbl[], dbl[]}[])
        n191 = property on="PltScanningPosition" class="XYGraph (strict)"(error in=w326) -> (error out=w325:errorcluster, "CrsrList"=w344:T8)  [unwired: 1 in, 1 out]
        n192 = Index Array(array=w344, index #1=0 ("index"), index #2=1 ("index")) -> (element #1=w341:T9, element #2=w340:T9)
        n193 = Index Array(array=w324, index=0) -> (element=w323:cluster{dbl[], dbl[]})
        n194 = Unbundle By Name(w341) -> ("Position.X"=w339:dbl)
        n195 = Unbundle By Name(w340) -> ("Position.X"=w336:dbl)
        n196 = Unbundle(w323) -> (w338:dbl[], w337:dbl[])
        n197 = Search 1D Array(1D array=w338, element=w339) -> (index of element=w335:i32)  [unwired: 1 in]
        n198 = Search 1D Array(1D array=w338, element=w336) -> (index of element=w334:i32)  [unwired: 1 in]
        n199 = Max & Min(x=w335, y=w334) -> (max(x,y)=w333:i32, min(x,y)=w332:i32)
        n200 = Subtract(x=w333, y=w332) -> (x-y=w331:i32)
        n201 = Increment(x=w331) -> (x+1=w330:i32)
        n202 = Array Subset(array=w337, index=w332, length=w330) -> (w329:dbl[])
        n203 = call <vilib>:"Std Deviation and Variance.vi"("X"=w329) -> ("mean"=→"SurfaceLevel":dbl, "standard deviation"=→"SurfaceError":dbl)  [unwired: 1 in, 1 out]
      }
      event "btnCalculateSlope": Value Change {
        w354 = T10 0 items=["Least Square", "Least Absolute Residual", "Bisquare"] ("method")
        n204 = event-data() -> ()  [unwired: 1 in, 5 out]
        n205 = local read "PltScanningPosition"() -> (w348:cluster{dbl[], dbl[]}[])
        n206 = property on="PltScanningPosition" class="XYGraph (strict)"(error in=w350) -> (error out=w349:errorcluster, "CrsrList"=w371:T8)  [unwired: 1 in, 1 out]
        n207 = Index Array(array=w371, index #1=0 ("index"), index #2=1 ("index")) -> (element #1=w368:T9, element #2=w367:T9)
        n208 = Index Array(array=w348, index=0) -> (element=w347:cluster{dbl[], dbl[]})
        n209 = Unbundle By Name(w368) -> ("Position.X"=w366:dbl)
        n210 = Unbundle By Name(w367) -> ("Position.X"=w364:dbl)
        n211 = Unbundle(w347) -> (w359:dbl[], w365:dbl[])
        n212 = Search 1D Array(1D array=w359, element=w366) -> (index of element=w363:i32)  [unwired: 1 in]
        n213 = Search 1D Array(1D array=w359, element=w364) -> (index of element=w362:i32)  [unwired: 1 in]
        n214 = Max & Min(x=w363, y=w362) -> (max(x,y)=w361:i32, min(x,y)=w357:i32)
        n215 = Subtract(x=w361, y=w357) -> (x-y=w360:i32)
        n216 = Increment(x=w360) -> (x+1=w358:i32)
        n217 = Array Subset(array=w359, index=w357, length=w358) -> (w355:dbl[])
        n218 = Array Subset(array=w365, index=w357, length=w358) -> (w356:dbl[])
        n219 = call <vilib>:"Linear Fit.vi"("Y"=w356, "X"=w355, "method"=w354) -> ("slope"=w352:dbl, "residue"=→"SlopeError":dbl)  [unwired: 8 in, 3 out]
        n220 = Reciprocal(x=w352) -> (1/x=→"Slope":dbl)
      }
    }
  }
  "error out" <- w7
  "PhaseRb" <- "Phase"
